vi "Car Wash Timer.vi"(3 "error in (no error)":errorcluster, 4 "Reset":bool, 5 "Controller":bool, 6 "Time":dbl) -> (0 "error out":errorcluster, 1 "Elapsed":bool, 2 "Elapsed Time":dbl)   [LabVIEW 2021]
panel:
  # "Timer"
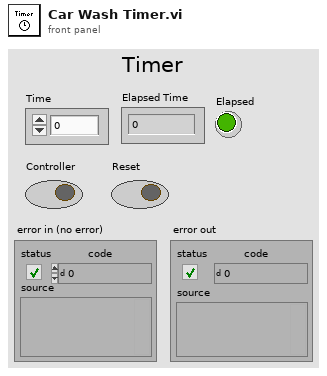
[diagram p1: front panel]
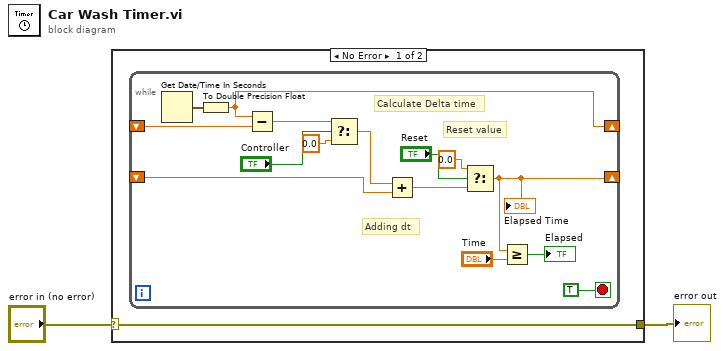
[diagram p0: block diagram]
diagram:
  n1 = case shown="No Error" "error in (no error)" {
    selector: "error in (no error)" -> [w3 w19]
    tunnel: [w3 w19] -> w1
    frame No Error {
      n2 = while {
        shift-right: [w16] -> _
        shift-left: _ -> [w17]
        shift-right: [w6] -> _
        shift-left: _ -> [w11]
        stop <- TRUE stop-if-true
        # "Reset value"
        # "Adding dt"
        # "Calculate Delta time"
        n3 = Get Date/Time In Seconds() -> (seconds since 1Jan1904=w18:timestamp)
        n4 = To Double Precision Float(number=w18) -> (double precision float=w16:dbl)
        n5 = Subtract(x=w16, y=w17) -> (x-y=w15:dbl)
        n6 = Select(t=w15, s="Controller", f=0.0) -> (s? t:f=w12:dbl)
        n7 = Add(x=w12, y=w11) -> (x+y=w10:dbl)
        n8 = Select(t=0.0, s="Reset", f=w10) -> (s? t:f=w6:dbl)
        "Elapsed Time" <- w6
        n9 = Greater Or Equal?(x=w6, y="Time") -> (x >= y?=→"Elapsed":bool)
      }
    }
    frame Error {
    }
  }
  "error out" <- w1
